vi "ReadDallasDS18B20.vi"(8 "error In":errorcluster, 11 "Select Com Port":refnum<visa-resource-name>) -> (0 "error Out":errorcluster, 1 "Temp in C (Number)":dbl, 2 "Temp in C (String)":string, 3 "return count":u32)   [LabVIEW 2020]
uses:
  <vilib>/Instr/_visa.llb/VISA Set IO Buffer Mask.ctl
  <vilib>/Instr/_visa.llb/VISA Configure Serial Port (Instr).vi
panel:
  out "Output String":string
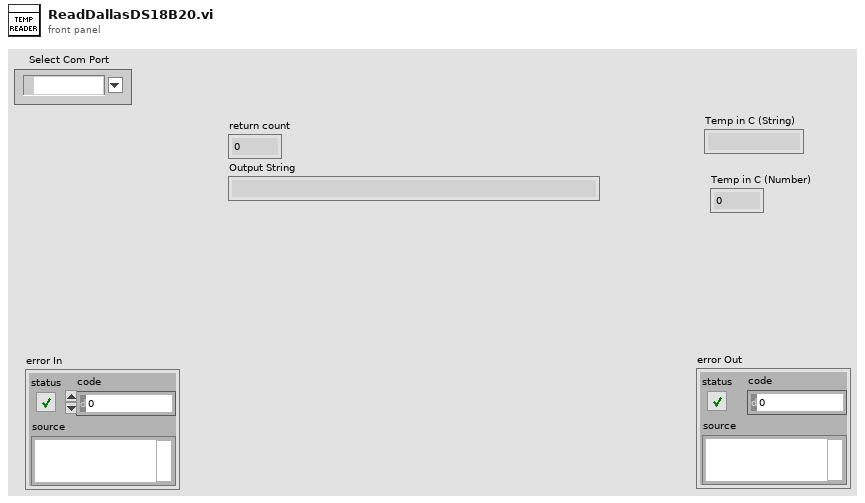
[diagram p1: front panel]
types:
  T1 = enum16{"Native", "Native Command Line", "UNIX", "Macintosh", "DOS"}
  T2 = typedef "VISA Set IO Buffer Mask.ctl" = u16
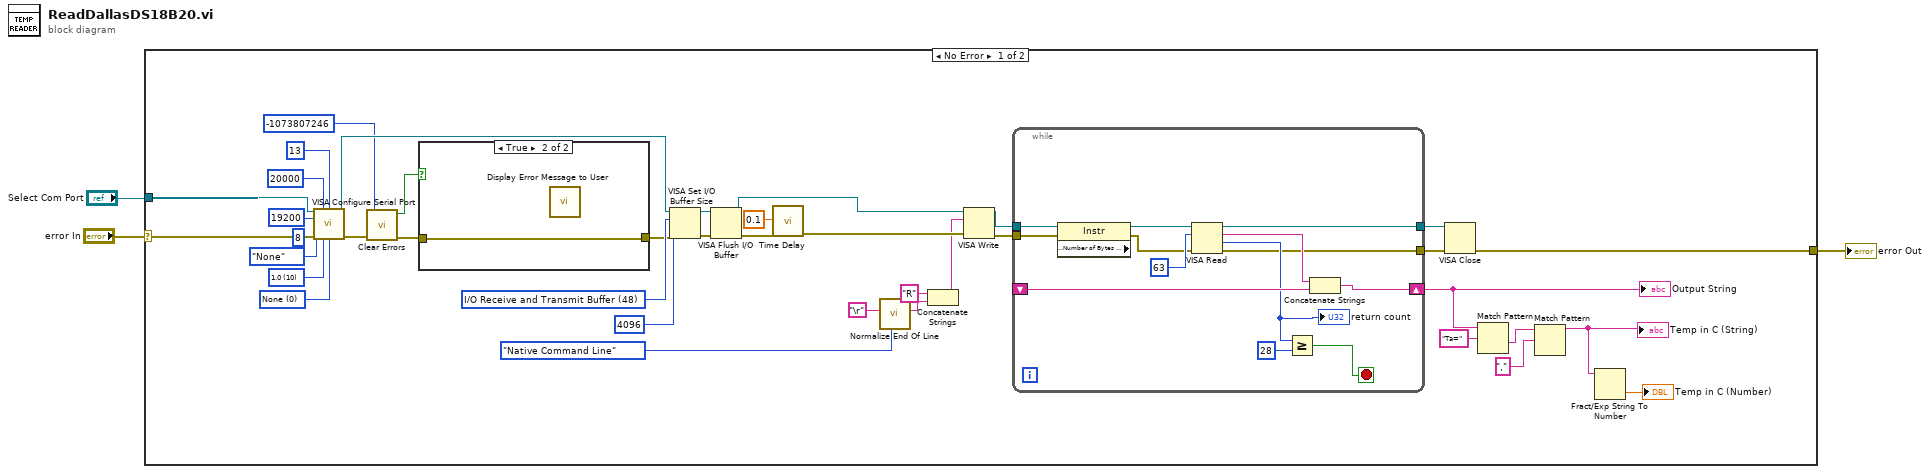
[diagram p0: block diagram]
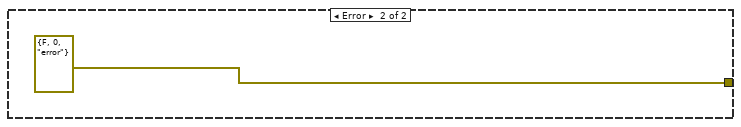
[diagram p3: hidden frame]
diagram:
  n1 = case shown="No Error" "error In" {
    selector: "error In" -> [w42 _]
    tunnel: [w18 errorcluster {"status"=FALSE, "code"=0, "source"="error"} ("error IO")] -> w2
    tunnel: "Select Com Port" -> [w41 _]
    frame No Error {
      w32 = T2 48 items=["I/O Receive Buffer"=16, "I/O Transmit Buffer"=32, "I/O Receive and Transmit Buffer"=48] ("Mask")
      w36 = u16 0 items=["None", "XON/XOFF", "RTS/CTS", "XON/XOFF & RTS/CTS", "DTR/DSR", "XON/XOFF & DTR/DSR"] ("flow control (0:none)")
      w37 = u16 10 items=["1.0"=10, "1.5"=15, "2.0"=20] ("stop bits (10: 1 bit)")
      n2 = call-poly "VISA Configure Serial Port"("VISA resource name"=w41, "timeout (10sec)"=u32 20000, "termination char\n(0xA = '\\n' = LF)"=u8 13 ("termination char\n(0xA = '\\n' = LF)"), "baud rate (9600)"=u32 19200, "data bits (8)"=u16 8, "parity (0:none)"=enum16{"None", "Odd", "Even", "Mark", "Space"}."None", "error in (no error)"=w42, "stop bits (10: 1 bit)"=w37, "flow control (0:none)"=w36) -> ("VISA resource name out"=w35:refnum<visa-resource-name>, "error out"=w12:errorcluster)  [unwired: 5 in]
      n3 = call <vilib>:"Clear Errors.vi"("error in (no error)"=w12, "specific error code to clear (0: all)"=-1073807246) -> ("error out"=w11:errorcluster, "specific error cleared?"=w10:bool)  [unwired: 4 in]
      n4 = case shown="True" w10 {
        tunnel: [w43 w44] -> w14
        tunnel: w11 -> [w43 w44]
        frame False {
        }
        frame True {
          n5 = call "Display Error Message to User"() -> ()  [unwired: 10 in, 2 out]
        }
      }
      n6 = VISA Set I/O Buffer Size(VISA resource name=w35, mask (16)=w32, size (4096)=u32 4096, error in (no error)=w14) -> (VISA resource name out=w33:refnum<visa-resource-name>, error out=w34:errorcluster)
      n7 = VISA Flush I/O Buffer(VISA resource name=w33, error in (no error)=w34) -> (VISA resource name out=w29:refnum<visa-resource-name>, error out=w30:errorcluster)  [unwired: 1 in]
      n8 = call "Time Delay"("error in (no error)"=w30, "Delay Time (s)"=0.1) -> ("error out"=w28:errorcluster)  [unwired: 9 in]
      n9 = call <vilib>:"Normalize End Of Line.vi"("end of line (Native)"=T1."Native Command Line", "string in"="\r") -> ("string out"=w27:string)  [unwired: 6 in]
      n10 = Concatenate Strings("R" ("string"), w27) -> (w23:string)
      n11 = VISA Write(VISA resource name=w29, write buffer=w23, error in (no error)=w28) -> (VISA resource name out=w21:refnum<visa-resource-name>, error out=w22:errorcluster)  [unwired: 1 out]
      n12 = while {
        tunnel: w22 -> [w57]
        tunnel: w21 -> [w56]
        shift-right: [w48] -> w9
        shift-left: _ -> [w49]
        tunnel: [w46] -> w20
        tunnel: [w45] -> w19
        stop <- w52 stop-if-true
        n13 = property class="Instr" props=["Serial Settings:Number of Bytes at Serial Port"](reference=w56, error in=w57) -> (reference out=w55:refnum<visa-resource-name>, error out=w53:errorcluster)  [unwired: 1 out]
        n14 = VISA Read(VISA resource name=w55, byte count=u32 63, error in (no error)=w53) -> (VISA resource name out=w46:refnum<visa-resource-name>, read buffer=w50:string, return count=w47:u32, error out=w45:errorcluster)
        "return count" <- w47
        n15 = Greater Or Equal?(x=w47, y=u32 28) -> (x >= y?=w52:bool)
        n16 = Concatenate Strings(w50, w49) -> (w48:string)
      }
      "Output String" <- w9
      n17 = VISA Close(VISA resource name=w20, error in (no error)=w19) -> (error out=w18:errorcluster)
      n18 = Match Pattern(string=w9, regular expression="Ta=") -> (after substring=w7:string)  [unwired: 1 in, 3 out]
      n19 = Match Pattern(string=w7, regular expression=",") -> (before substring=w5:string)  [unwired: 1 in, 3 out]
      "Temp in C (String)" <- w5
      n20 = Fract/Exp String To Number(string=w5) -> (number=→"Temp in C (Number)":dbl)  [unwired: 3 in, 1 out]
    }
    frame Error {
    }
  }
  "error Out" <- w2
